vi "sub_load_DMD_mov_ext_trig.vi"(3 "SequenceRepeats":i32=1, 4 "binary mov path":path=path "C:/Users/cohen_lab/Desktop/Labview_code/DMD_control/DMD6images.bin") -> (0 "SequID":u32, 1 "DeviceID":u32, 2 "DevInq1":errorcluster)   [LabVIEW 2013]
uses:
  C:/Program Files/ALP-4.1/ALP-4.1 high-speed API/Samples/alpD41.dll
panel:
  in  "Exposure (us)":i32=1000
  out "Dev Control Error":errorcluster
  out "Labview":errorcluster
  out "SeqControl3":errorcluster
  out "PicNum":i32
  out "ProjStartErr":i32
  out "SeqPutErr":i32
  out "SeqControl1":errorcluster
  out "SeqControl2":errorcluster
  out "ProjControl":errorcluster
  out "SeqAllocErr":i32
  out "DevInq2":errorcluster
  out "DevAllocErr":i32
  out "DMD Type":string
  out "SerialNumber":i32
  # "Initialization"
  # "0 = no error"
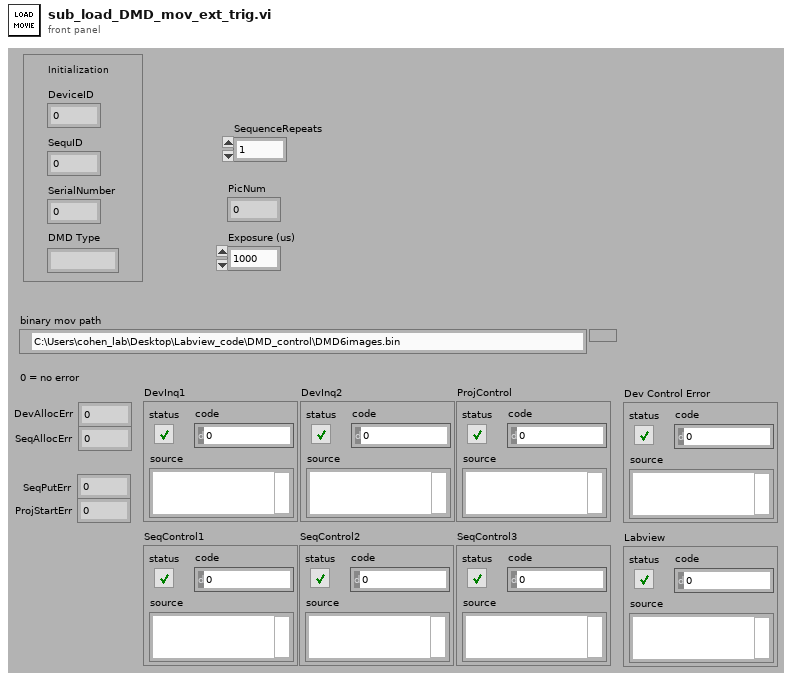
[diagram p1: front panel]
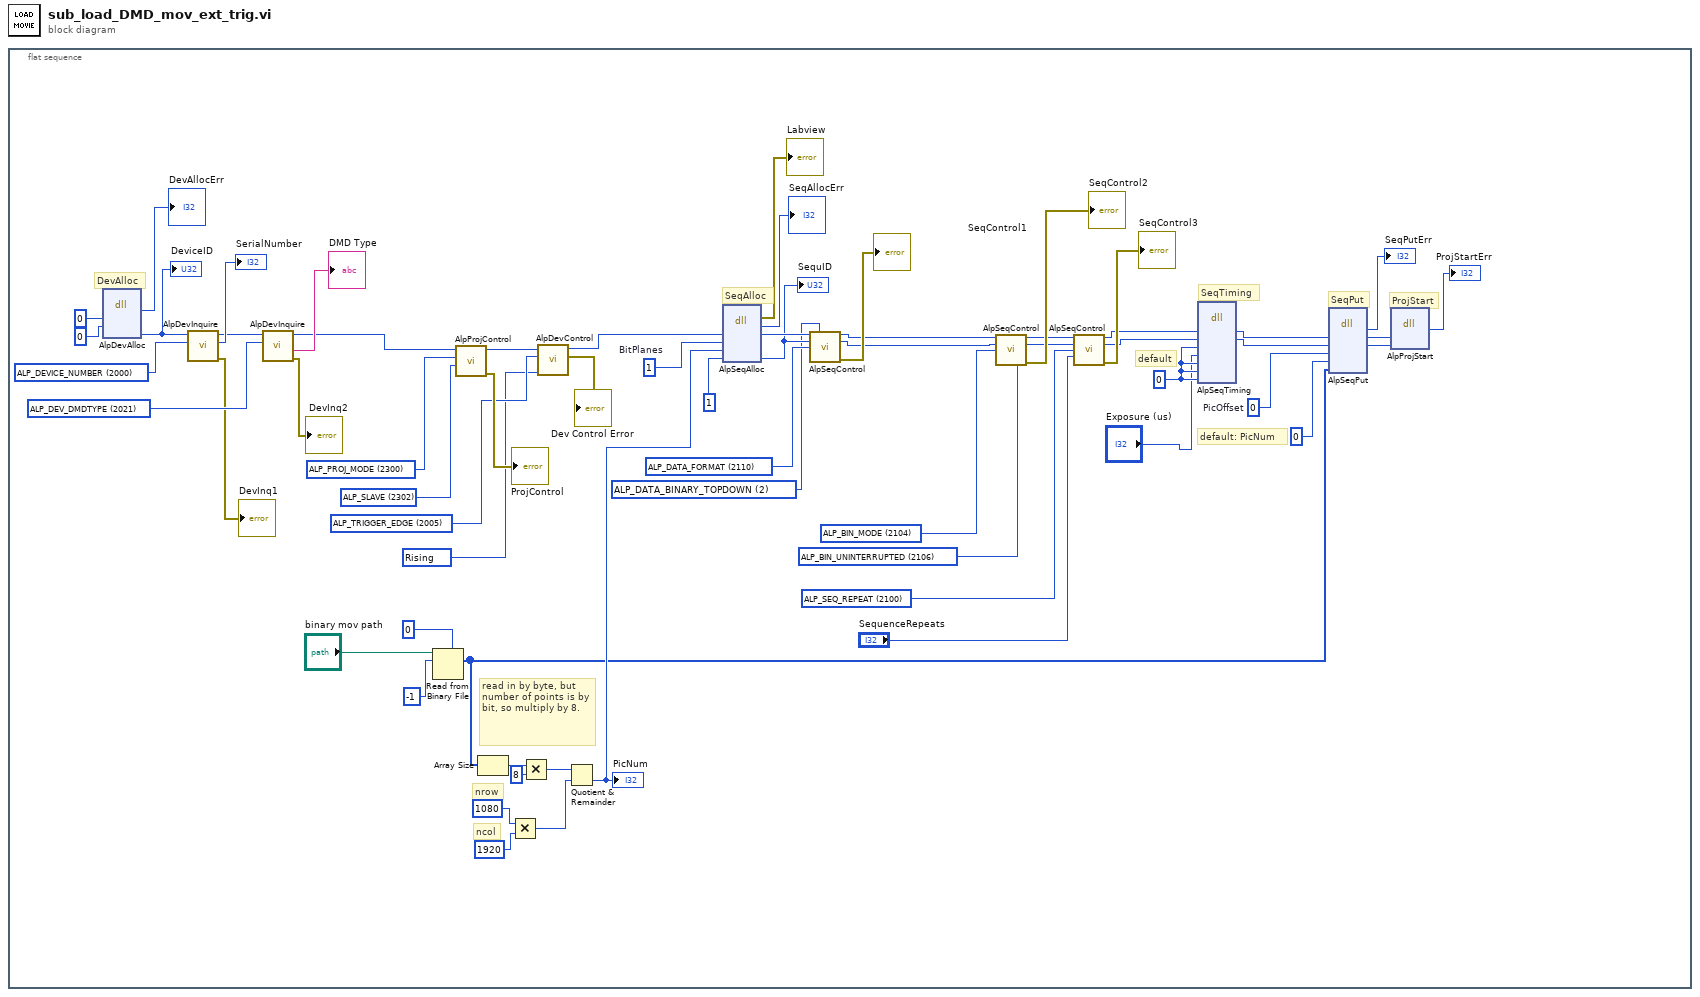
[diagram p0: block diagram]
diagram:
  n1 = flat-sequence {
    frame #0 {
      w6 = 0
      w11 = 2009 items=["Rising"=2009, "Falling"=2008] ("Trigger_Edge")
      w12 = 2005 items=["ALP_DEVICE_NUMBER"=2000, "ALP_VERSION"=2001, "ALP_DEV_STATE"=2002, "ALP_AVAIL_MEMORY"=2003, "ALP_SYNCH_POLARITY"=2004, "ALP_TRIGGER_EDGE"=2005, "ALP_USB_CONNECTION"=2016, "ALP_DEV_DMDTYPE"=2021, "ALP_DEV_DISPLAY_HEIGHT"=2057, "ALP_DEV_DISPLAY_WIDTH"=2058, "ALP_PWM_LEVEL"=2063, "ALP_DEV_DMD_MODE"=2064] ("InquireType")
      w19 = 2100 items=["ALP_SEQ_REPEAT"=2100, "ALP_FIRSTFRAME"=2101, "ALP_LASTFRAME"=2102, "ALP_BITNUM"=2103, "ALP_BIN_MODE"=2104, "ALP_DATA_FORMAT"=2110, "ALP_SEQ_PUT_LOCK"=2119] ("ControlType")
      w36 = 2300 items=["ALP_PROJ_MODE"=2300, "ALP_PROJ_INVERSION"=2306, "ALP_PROJ_UPSIDE_DOWN"=2307] ("ControlType")
      w8 = 2302 items=["ALP_MASTER"=2301, "ALP_SLAVE"=2302] ("ProjectorMode")
      w42 = 2106 items=["ALP_BIN_NORMAL"=2105, "ALP_BIN_UNINTERRUPTED"=2106] ("Binary Mode")
      w43 = 2104 items=["ALP_SEQ_REPEAT"=2100, "ALP_FIRSTFRAME"=2101, "ALP_LASTFRAME"=2102, "ALP_BITNUM"=2103, "ALP_BIN_MODE"=2104, "ALP_DATA_FORMAT"=2110, "ALP_SEQ_PUT_LOCK"=2119] ("ControlType")
      w44 = 2 items=["ALP_DATA_MSB_ALIGN", "ALP_DATA_LSB_ALIGN", "ALP_DATA_BINARY_TOPDOWN", "ALP_DATA_BINARY_BOTTOMUP"] ("Data Format")
      w45 = 2110 items=["ALP_SEQ_REPEAT"=2100, "ALP_FIRSTFRAME"=2101, "ALP_LASTFRAME"=2102, "ALP_BITNUM"=2103, "ALP_BIN_MODE"=2104, "ALP_DATA_FORMAT"=2110, "ALP_SEQ_PUT_LOCK"=2119] ("ControlType")
      w48 = 0  # PicOffset
      w55 = 2021 items=["ALP_DEVICE_NUMBER"=2000, "ALP_VERSION"=2001, "ALP_DEV_STATE"=2002, "ALP_AVAIL_MEMORY"=2003, "ALP_SYNCH_POLARITY"=2004, "ALP_TRIGGER_EDGE"=2005, "ALP_USB_CONNECTION"=2016, "ALP_DEV_DMDTYPE"=2021, "ALP_DEV_DISPLAY_HEIGHT"=2057, "ALP_DEV_DISPLAY_WIDTH"=2058, "ALP_PWM_LEVEL"=2063, "ALP_DEV_DMD_MODE"=2064] ("InquireType")
      w57 = 2000 items=["ALP_DEVICE_NUMBER"=2000, "ALP_VERSION"=2001, "ALP_DEV_STATE"=2002, "ALP_AVAIL_MEMORY"=2003, "ALP_SYNCH_POLARITY"=2004, "ALP_TRIGGER_EDGE"=2005, "ALP_USB_CONNECTION"=2016, "ALP_DEV_DMDTYPE"=2021, "ALP_DEV_DISPLAY_HEIGHT"=2057, "ALP_DEV_DISPLAY_WIDTH"=2058, "ALP_PWM_LEVEL"=2063, "ALP_DEV_DMD_MODE"=2064] ("InquireType")
      w62 = 1  # BitPlanes
      # "default"
      # "SeqTiming"
      # "read in by byte, but number of points is by bit, so multiply by 8."
      # "nrow"
      # "ncol"
      # "default: PicNum"
      # "ProjStart"
      # "SeqPut"
      # "DevAlloc"
      # "SeqAlloc"
      n2 = dll-call lib="C:/Program Files/ALP-4.1/ALP-4.1 high-speed API/Samples/alpD41.dll" fn="AlpDevAlloc"("DeviceNum"=0, "InitFlag"=0) -> ("return type"=→"DevAllocErr":i32, "DeviceIdPtr"=w59:u32)  [unwired: 6 in, 2 out]
      "DeviceID" <- w59
      n3 = call "AlpDevInquire.vi"("InquireType"=w57, "DeviceID"=w59) -> ("Error OUT"=→"DevInq1":errorcluster, "Output Number"=→"SerialNumber":i32, "DeviceIDout"=w56:u32)  [unwired: 6 in, 1 out]
      n4 = call "AlpDevInquire.vi"("InquireType"=w55, "DeviceID"=w56) -> ("Error OUT"=→"DevInq2":errorcluster, "Output Text"=→"DMD Type":string, "DeviceIDout"=w7:u32)  [unwired: 6 in, 1 out]
      n5 = Read from Binary File(5:u8 0, 10:-1 ("count (1)"), 11:"binary mov path") -> (2:w26:u8[])  [unwired: 3 in, 3 out]
      n6 = call "AlpProjControl.vi"("ProjectorMode"=w8, "ControlType"=w36, "DeviceID"=w7) -> ("Error OUT"=→"ProjControl":errorcluster, "DeviceIDout"=w15:u32)  [unwired: 7 in]
      n7 = Array Size(array=w26) -> (size(s)=w24:i32)
      n8 = Multiply(x=1080, y=1920) -> (x*y=w29:i32)
      n9 = Multiply(x=w24, y=8) -> (x*y=w22:i32)
      n10 = call "AlpDevControl.vi"("Trigger_Edge"=w11, "InquireType"=w12, "DeviceID"=w15) -> ("Error OUT"=→"Dev Control Error":errorcluster, "DeviceId"=w13:u32)  [unwired: 7 in]
      n11 = Quotient & Remainder(x=w22, y=w29) -> (floor(x/y)=w27:i32)  [unwired: 1 out]
      "PicNum" <- w27
      n12 = dll-call lib="C:/Program Files/ALP-4.1/ALP-4.1 high-speed API/Samples/alpD41.dll" fn="AlpSeqAlloc"("DeviceId"=w13, "BitPlanes"=w62, "PicNum"=w27, "SequenceIdPtr"=u32 1) -> (error out=→"Labview":errorcluster, "return type"=→"SeqAllocErr":i32, "DeviceId"=w47:u32, "SequenceIdPtr"=w46:u32)  [unwired: 5 in, 1 out]
      "SequID" <- w46
      n13 = call "AlpSeqControl.vi"("DeviceID"=w47, "Data Format"=w44, "SequenceID"=w46, "ControlType"=w45) -> ("DeviceIDout"=w10:u32, "SequenceIDout"=w9:u32, "Error OUT"=→"SeqControl1":errorcluster)  [unwired: 9 in]
      n14 = call "AlpSeqControl.vi"("DeviceID"=w10, "SequenceID"=w9, "ControlType"=w43, "Binary Mode"=w42) -> ("DeviceIDout"=w21:u32, "SequenceIDout"=w20:u32, "Error OUT"=→"SeqControl2":errorcluster)  [unwired: 9 in]
      n15 = call "AlpSeqControl.vi"("DeviceID"=w21, "SequenceID"=w20, "ControlType"=w19, "SequenceRepeats"="SequenceRepeats") -> ("DeviceIDout"=w5:u32, "SequenceIDout"=w4:u32, "Error OUT"=→"SeqControl3":errorcluster)  [unwired: 9 in]
      n16 = dll-call lib="C:/Program Files/ALP-4.1/ALP-4.1 high-speed API/Samples/alpD41.dll" fn="AlpSeqTiming"("DeviceId"=w5, "SequenceId"=w4, "IlluminateTime"=w6, "PictureTime"="Exposure (us)", "TriggerDelay"=w6, "TriggerPulseWidth"=w6, "VdDelay"=w6) -> ("DeviceId"=w3:u32, "SequenceId"=w2:u32)  [unwired: 9 in, 2 out]
      n17 = dll-call lib="C:/Program Files/ALP-4.1/ALP-4.1 high-speed API/Samples/alpD41.dll" fn="AlpSeqPut"("DeviceId"=w3, "SequenceId"=w2, "PicOffset"=w48, "PicLoad"=0, "UserArrayPtr"=w26) -> ("return type"=→"SeqPutErr":i32, "DeviceId"=w39:u32, "SequenceId"=w38:u32)  [unwired: 6 in, 2 out]
      n18 = dll-call lib="C:/Program Files/ALP-4.1/ALP-4.1 high-speed API/Samples/alpD41.dll" fn="AlpProjStart" ("alpD40.dll:AlpProjStartCont")("DeviceId"=w39, "SequenceId"=w38) -> ("return type"=→"ProjStartErr":i32)  [unwired: 5 in, 2 out]
    }
  }
